vi "underscore_output.vi"() -> (3 "_status":dbl=42.0)   [LabVIEW 2020]
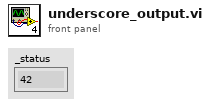
[diagram p1: front panel]
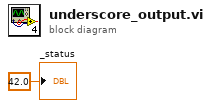
[diagram p0: block diagram]
diagram:
  "_status" <- 42.0
